vi "SampleClient.vi"() -> ()   [LabVIEW 2012]
doc: "A sample client that can be run on the computer or RIO"
panel:
  in  "Show Web":bool
  out "Answer":string
  in  "LED":bool
  out "time":string
  out "Status":string
  in  "stop":bool
  # "Instructions:\n1. Run the VI\n2. Verify that you see the correct time.\n3. Press the LED button. You should see the LED reply change.\nIf you are targetting a myRIO, the LED should change as well.\n4. Debug by clicking Show Webpage.\n5. See what is being sent back and forth by clicking Show Webpage."
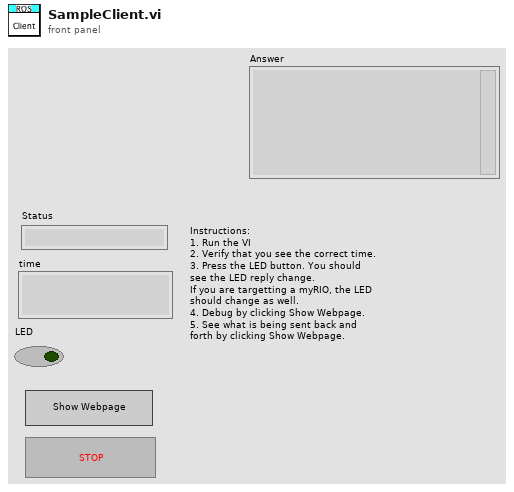
[diagram p1: front panel]
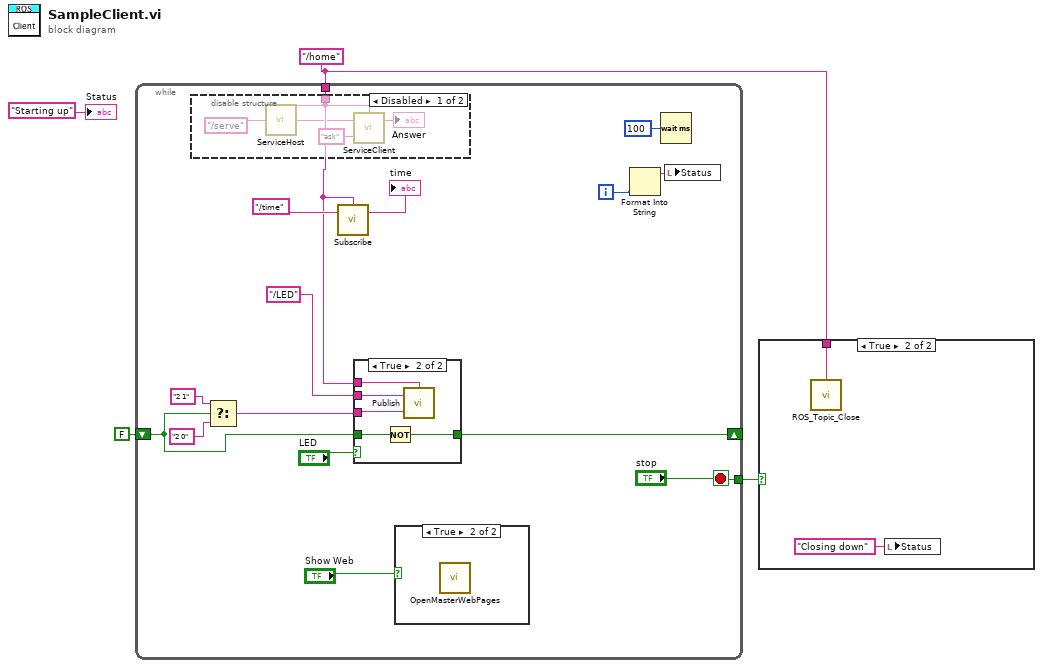
[diagram p0: block diagram]
diagram:
  w1 = "/home" ("Topic")
  n1 = while {
    tunnel: ["stop"] -> w2
    tunnel: w1 -> [w6]
    shift-right: [w13] -> _
    shift-left: FALSE -> [w12]
    i -> [w17]
    stop <- "stop" stop-if-true
    n2 = disable-structure shown="Disabled" {
      disable-tunnel: w6 -> [w27 _]
      frame Disabled {
        w26 = "/serve" ("Topic")
        n3 = call <userlib>:"ServiceHost.vi"("Topic"=w26, "node"=w27) -> ()  [unwired: 1 in, 2 out]
        n4 = call <userlib>:"ServiceClient.vi"("Msg in"="ask", "Topic"=w26, "node"=w27) -> ("Reply"=→"Answer":string)  [unwired: 1 out]
      }
      frame Enabled {
      }
    }
    n5 = Select(t="2 1" ("Status"), s=w12, f="2 0" ("Status")) -> (s? t:f=w14:string)
    n6 = call <userlib>:"Subscribe.vi"("Topic"="/time", "node"=w6) -> ("Reply"=→"time":string)  [unwired: 1 in, 1 out]
    n7 = case shown="True" "LED" {
      tunnel: w6 -> [_ w21]
      tunnel: "/LED" ("Topic") -> [_ w22]
      tunnel: w14 -> [_ w23]
      tunnel: [w20 w24] -> w13
      tunnel: w12 -> [w20 w25]
      frame False {
      }
      frame True {
        n8 = Not(x=w25) -> (.not. x?=w24:bool)
        n9 = call <userlib>:"Publish.vi"("String"=w23, "Topic"=w22, "node"=w21) -> ()  [unwired: 1 in, 1 out]
      }
    }
    n10 = case shown="True" "Show Web" {
      frame False {
      }
      frame True {
        n11 = call <userlib>:"OpenMasterWebPages.vi"() -> ()  [unwired: 4 in]
      }
    }
    n12 = Format Into String(w17) -> (resulting string=w18:string)  [unwired: 3 in, 1 out]
    n13 = Wait (ms)(milliseconds to wait=u32 100) -> ()  [unwired: 1 out]
    n14 = local write "Status"(w18) -> ()
  }
  n15 = case shown="True" w2 {
    tunnel: w1 -> [_ w30]
    frame False {
    }
    frame True {
      n16 = call <userlib>:"ROS_Topic_Close.vi"("node"=w30) -> ()  [unwired: 3 in, 1 out]
      n17 = local write "Status"("Closing down" ("Status")) -> ()
    }
  }
  "Status" <- "Starting up" ("Status")
